vi "Auto_Inspection Station MainS8.vi"(7 "Boolean 2":refnum<vi>, 8 "站別":refnum<vi>, 9 "站別":i32, 10 "ActRef":refnum<vi>, 11 "Station Action.lvclass":refnum<class "Station Action.lvclass">) -> ()   [LabVIEW 2019]
uses:
  Station Class/Station Action.lvclass
  Ctrl/Station Action.ctl
  Ctrl/Auto Inspection Data Name.ctl
  FlowCtrl Class/Ctrl/Auto Inspection_IN Name2.ctl
  FlowCtrl Class/Vision AI/Ctl/S8 Station IO.ctl
  Ctrl/ModbusCmd.ctl
  Function/Main UI/Glb/Main_UI Gb.vi
  LLB/Commonly VI/Main Glb.vi
  Ctrl/Auto Inspection Main UI Ref.ctl
  LLB/Commonly VI.lvlib
  Ctrl/Auto Inspection Station Name2.ctl
panel:
  in  "Boolean":bool
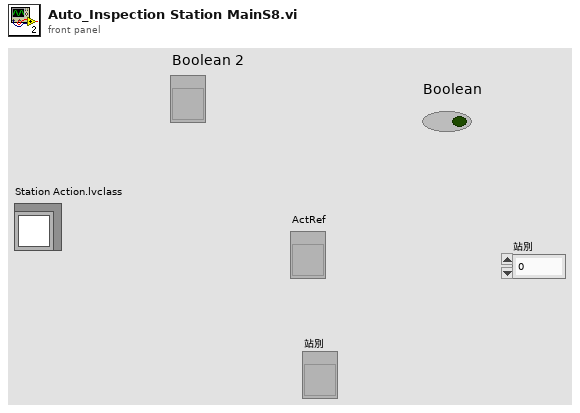
[diagram p1: front panel]
types:
  T1 = typedef "Station Action.ctl" = enum16{"Wait Item In", "Dectect Action", "ImformOut"}
  T2 = cluster{"AutoRunFlg":refnum<vi>, "Action Finish Flg":refnum<vi>, "Remaining Action":refnum<vi>, "Btn_AutoRun":refnum<vi>, "Manual Flg":refnum<vi>, "Sub Process Error":refnum<vi>}
  T3 = typedef "Auto Inspection Data Name.ctl" = enum16{"LocalRun", "ItemSN(TimeCode)", "CurrentAction", "Error", "Data", "OKNG", "電壓值", "電壓值判斷", "電流值", "電流值判斷", "Laser1 Data", "Laser2 Data", "Laser OKNG", "StationNO"}
  T4 = cluster{"starting address":u16, "number of inputs":u16, "Sat Coils":bool[], "Holding Registers":u16[]}
  T5 = typedef "ModbusCmd.ctl" = enum16{"Connect", "Disconnect", "Init", "Fetch Basic Objects", "Fetch Input Refisters", "Fetch Discrete Inputs", "Set Coils", "Set Holding Registers", "Write Single Holding", "Exit"}
  T6 = typedef "Auto Inspection_IN Name2.ctl" = enum16{"S0 Station", "S1 Barcode ", "S2 Tool Format", "S3 Tool Prpgram", "S4 Tool Sacn", "S11 Laser Detect", "S8 Vision AI"}
  T7 = typedef "S8 Station IO.ctl" = enum16{"S8_PC動作中(address 80)", "S8 AI 浪代OK(address 81)", "S8 AI 浪代NG(address 82)", "S8 AI 動作完成"}
  T8 = typedef "Auto Inspection Station Name2.ctl" = enum16{"S1Barcode", "S2Measure", "S3Measure", "S4Measure", "S5Measure", "S11_LaserCheck", "S8_Vision AI"}
  T9 = typedef "Auto Inspection Main UI Ref.ctl" = cluster{"LineScan arrive":refnum<vi>, "LineScanfinish":refnum<vi>, "AI arrive":refnum<vi>, "AI finish":refnum<vi>, "NG Pick arrive":refnum<vi>, "NG Pick finish":refnum<vi>}
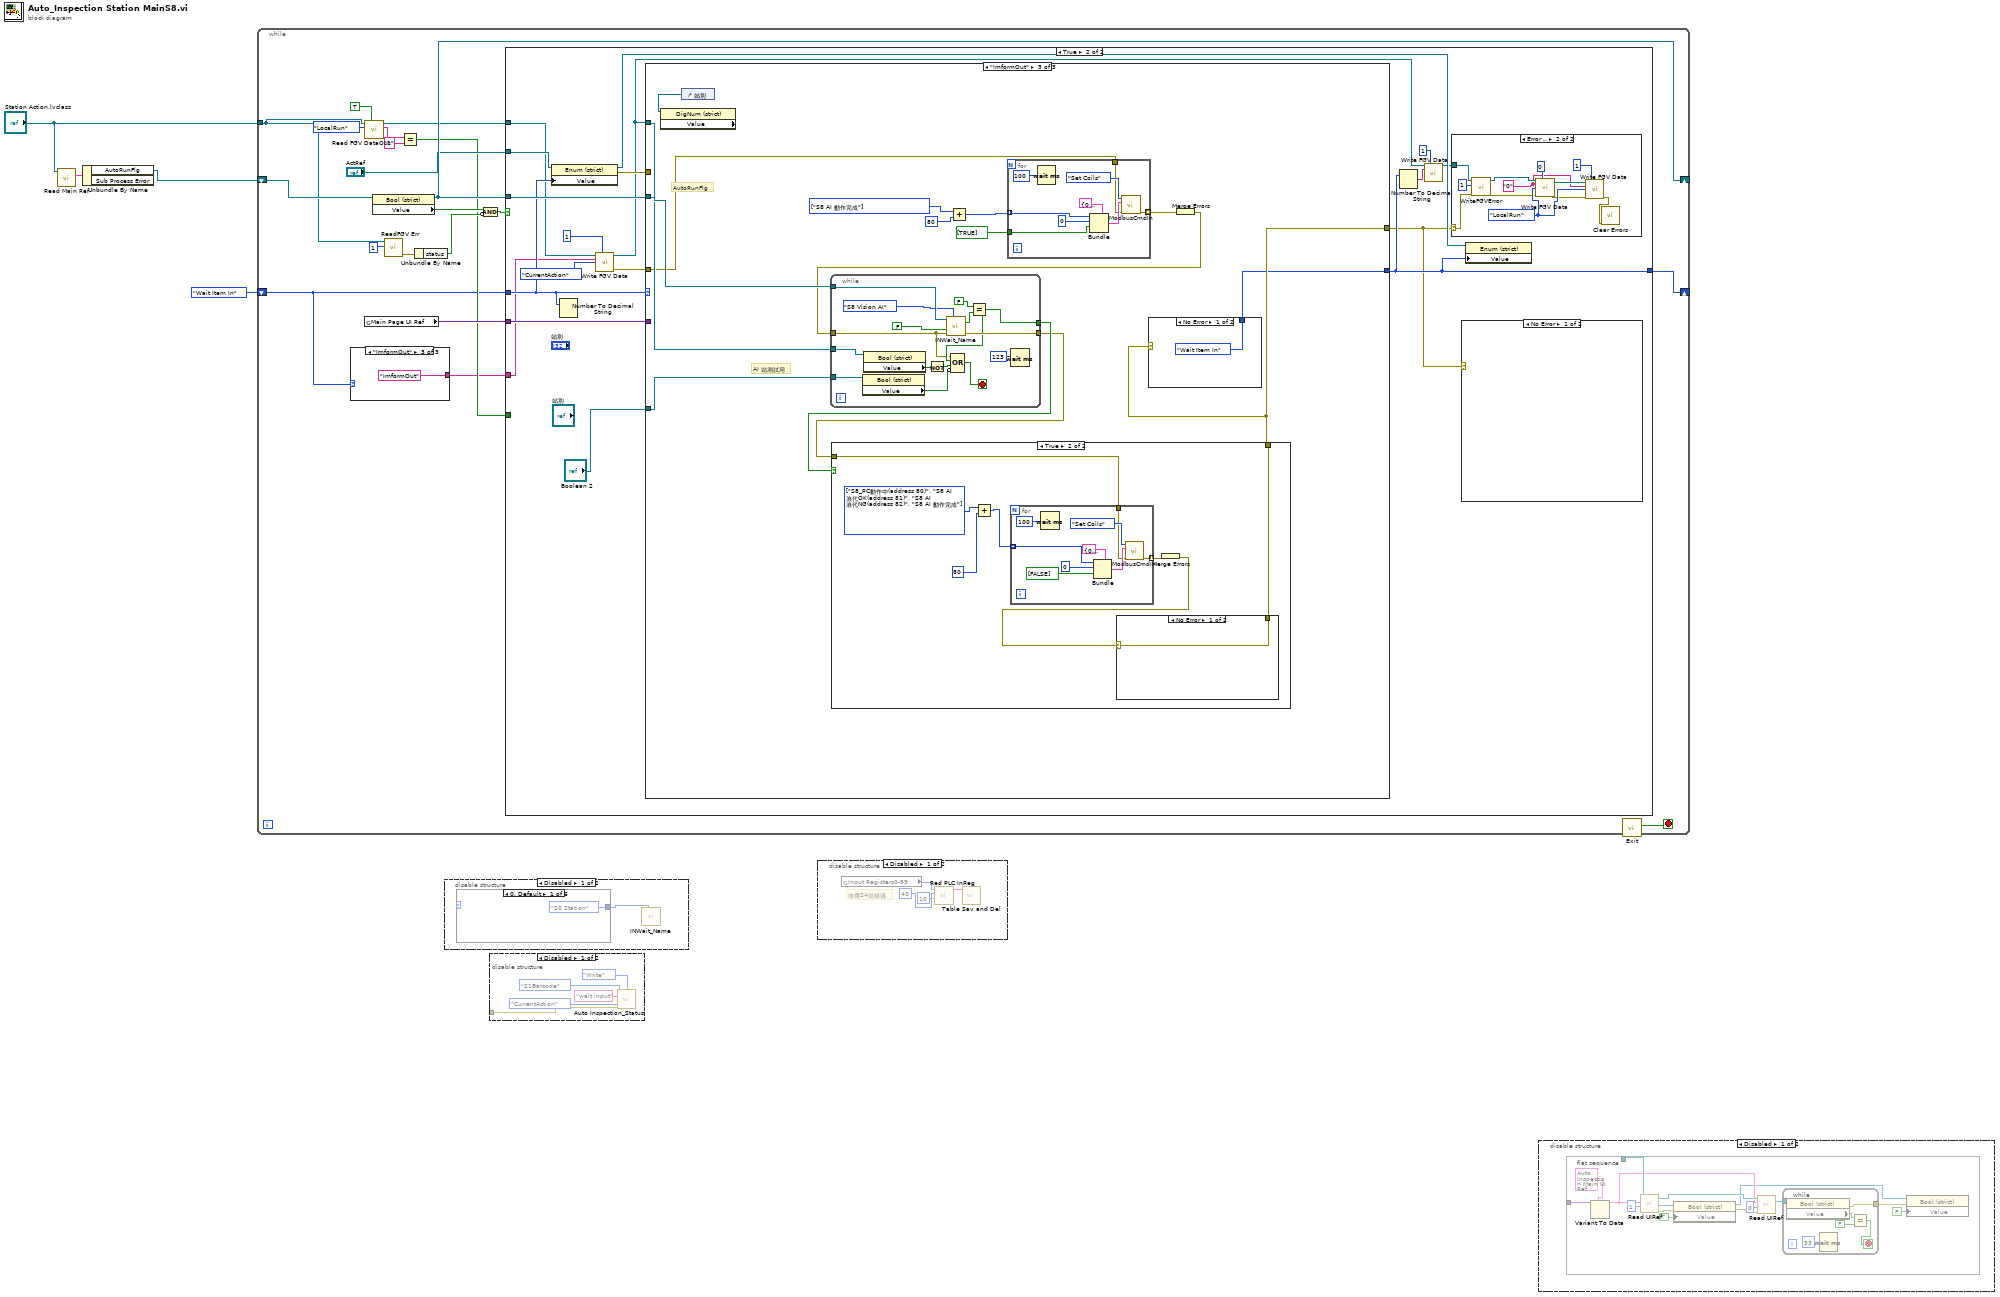
[diagram p0: block diagram]
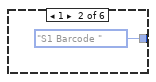
[diagram p3: hidden frame]
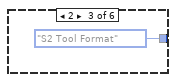
[diagram p4: hidden frame]
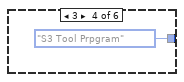
[diagram p5: hidden frame]
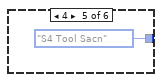
[diagram p6: hidden frame]
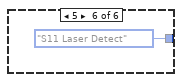
[diagram p7: hidden frame]
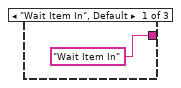
[diagram p11: hidden frame]
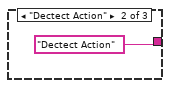
[diagram p12: hidden frame]
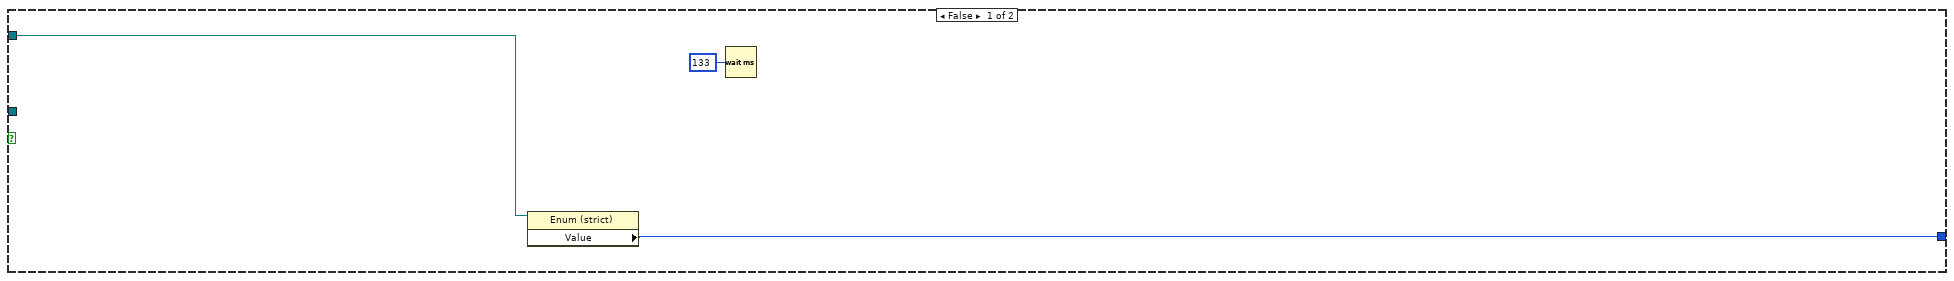
[diagram p13: hidden frame]
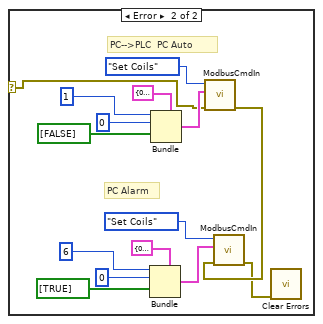
[diagram p14: hidden frame]
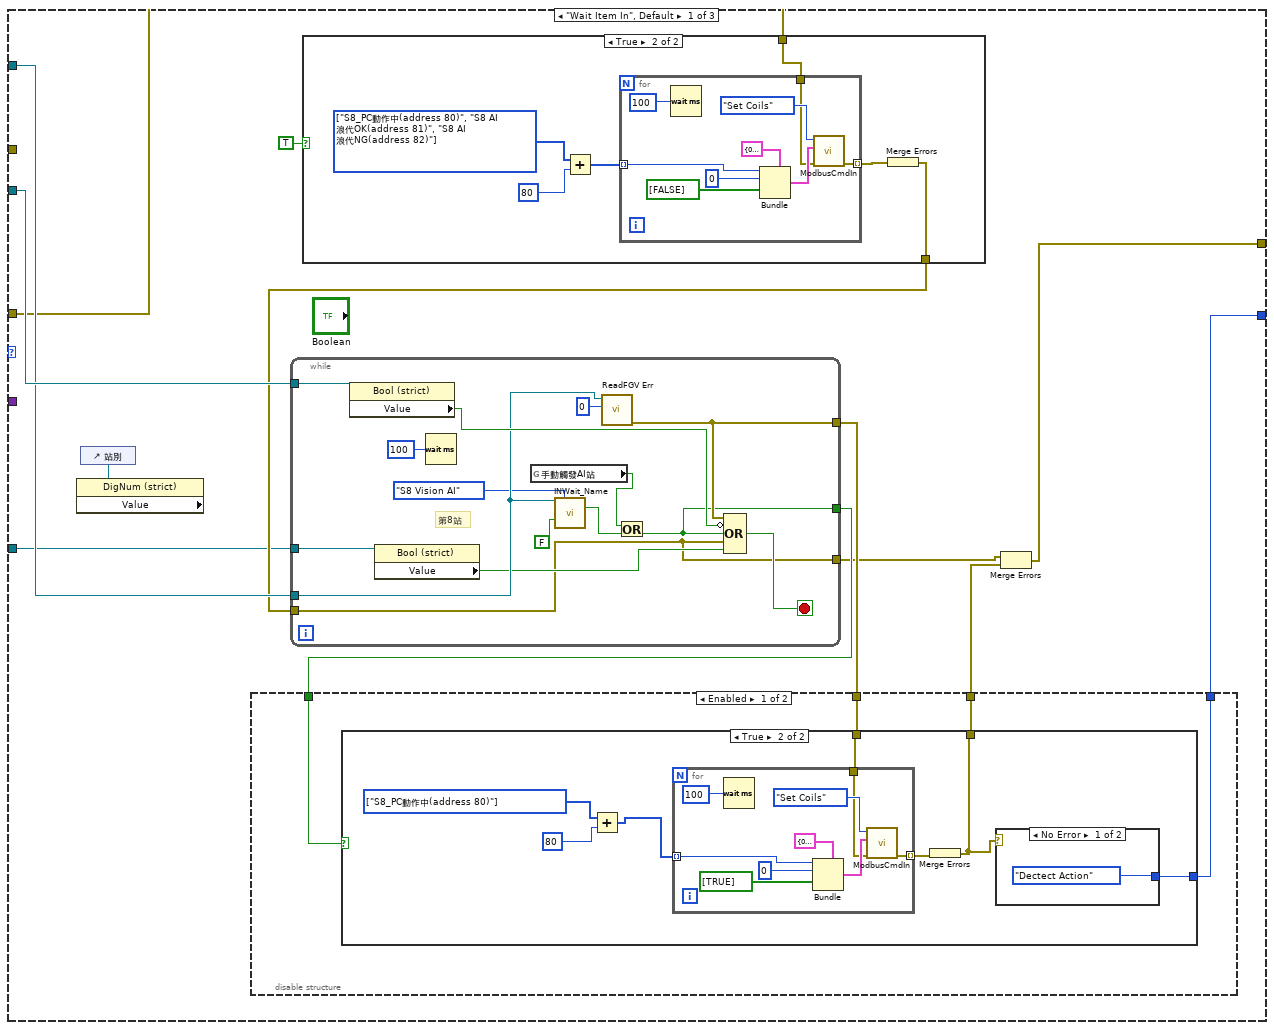
[diagram p16: hidden frame]
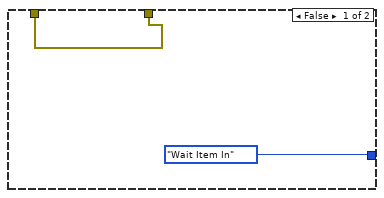
[diagram p17: hidden frame]
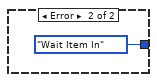
[diagram p18: hidden frame]
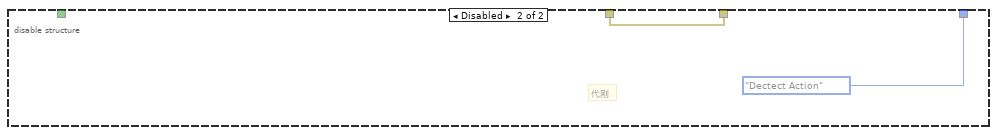
[diagram p19: hidden frame]
diagram:
  n1 = call-dynamic "Read Main Ref.vi"("Main Process Class in"="Station Action.lvclass") -> ("Main Ref"=w3:T2)  [unwired: 8 in, 2 out]
  n2 = Unbundle By Name(w3) -> ("AutoRunFlg"=w1:refnum<vi>)  [unwired: 1 out]
  n3 = while {
    shift-right: [w20] -> _
    shift-left: Station_Action."Wait Item In" -> [w6]
    tunnel: "Station Action.lvclass" -> [w8]
    shift-right: [w18] -> _
    shift-left: w1 -> [w23]
    stop <- w19 stop-if-true
    n4 = case shown="\"ImformOut\"" w6 {
      tunnel: ["Wait Item In" "Dectect Action" "ImformOut"] -> w5
      frame "Wait Item In", Default {
      }
      frame "Dectect Action" {
      }
      frame "ImformOut" {
      }
    }
    n5 = call-dynamic "Read FGV DataOut.vi"("TSt/FConveyor"=TRUE, "Data"=Auto_Inspection_Data_Name."LocalRun", "Station Action in"=w8) -> ("DataOut"=w11:string, "Station Action out"=w14:refnum<class "Station Action.lvclass">)  [unwired: 6 in, 1 out]
    n6 = global read "Main_UI Gb.vi" "Main Page UI Ref"() -> (w21:variant)
    n7 = property class="Bool (strict)"(reference=w23) -> (reference out=w18:refnum<vi>, "Value"=w24:bool)  [unwired: 1 in, 1 out]
    n8 = call-dynamic "ReadFGV Err.vi"("0Cv/1ST"=1, "Station Action in"=w8) -> ("error out"=w16:errorcluster)  [unwired: 8 in, 1 out]
    n9 = Equal?(x=w11, y="1") -> (x = y?=w7:bool)
    n10 = Unbundle By Name(w16) -> ("status"=w15:bool)
    n11 = Compound Arithmetic op=AND(w24, invert w15) -> (w22:bool)
    n12 = case shown="True" w22 {
      tunnel: w18 -> [_ w47]
      tunnel: w6 -> [_ w40]
      tunnel: w21 -> [_ w48]
      tunnel: w14 -> [_ w34]
      tunnel: [w29 w37] -> w20
      tunnel: "ActRef" -> [w30 w46]
      tunnel: w7 -> [_ _]
      tunnel: w5 -> [_ w33]
      frame False {
        n13 = property class="Enum (strict)"(reference=w30) -> ("Value"=w29:T1)  [unwired: 1 in, 2 out]
        n14 = Wait (ms)(milliseconds to wait=u32 133) -> ()  [unwired: 1 out]
      }
      frame True {
        n15 = property class="Enum (strict)"(reference=w46, "Value"=w40) -> (reference out=w45:refnum<vi>, error out=w44:errorcluster)  [unwired: 1 in]
        n16 = Number To Decimal String(number=w40) -> ()  [unwired: 1 in, 1 out]
        n17 = call-dynamic "Write FGV Data.vi"("Station Action in"=w34, "0Cv/1St"=1, "DataIn"=w33, "Data"=Auto_Inspection_Data_Name."CurrentAction") -> ("Station Action out"=w36:refnum<class "Station Action.lvclass">, "error out"=w41:errorcluster)  [unwired: 10 in]
        n18 = case shown="\"ImformOut\"" w40 {
          tunnel: w48 -> [_ _ _]
          tunnel: w36 -> [w87 w148 w165]
          tunnel: w47 -> [w88 _ w164]
          tunnel: [w85 w146 w160] -> w37
          tunnel: w44 -> [_ _ _]
          tunnel: [w77 w147 w161] -> w31
          tunnel: w41 -> [w84 _ w163]
          tunnel: "Boolean 2" -> [w80 _ w151]
          frame "Wait Item In", Default {
            n19 = control-ref of="站別"() -> (w86:refnum<vi>)
            n20 = property class="DigNum (strict)" props=["Value"](reference=w86) -> ()  [unwired: 1 in, 3 out]
            n21 = case shown="True" TRUE {
              tunnel: w84 -> [w115 w121]
              tunnel: [w115 w118] -> w82
              frame False {
                # "代刚"
              }
              frame True {
                w116 = T7[] [enum."S8_PC動作中(address 80)", enum."S8 AI 浪代OK(address 81)", enum."S8 AI 浪代NG(address 82)"] items=["S8_PC動作中(address 80)", "S8 AI 浪代OK(address 81)", "S8 AI 浪代NG(address 82)", "S8 AI 動作完成"]
                n22 = Add(x=w116, y=80) -> (x+y=w120:i32[])
                n23 = for {
                  tunnel: [w124] -> w117 mode=indexing
                  tunnel: w120 -> [w123] mode=indexing
                  tunnel: w121 -> [w122]
                  n24 = Wait (ms)(milliseconds to wait=100) -> ()  [unwired: 1 out]
                  n25 = Bundle(cluster=T4 {"starting address"=0, "number of inputs"=0, "Sat Coils"=[], "Holding Registers"=[]} ("data"), "starting address"=w123, "number of inputs"=u16 0, "Sat Coils"=bool[] [FALSE]) -> (w127:T4)  [unwired: 1 in]
                  n26 = call "ModbusCmdIn.vi"("error in (no error)"=w122, "data"=w127, "Enum"=ModbusCmd."Set Coils") -> ("error out"=w124:errorcluster)  [unwired: 8 in]
                }
                n27 = Merge Errors(w117) -> (w118:errorcluster)
              }
            }
            n28 = while {
              tunnel: [w141] -> w83
              tunnel: w82 -> [w133]
              tunnel: [w132] -> w81
              tunnel: w87 -> [w137]
              tunnel: w88 -> [w138]
              tunnel: w80 -> [w135]
              tunnel: [w133] -> w79
              stop <- w145 stop-if-true
              # "第8站"
              n29 = property class="Bool (strict)"(reference=w138) -> ("Value"=w143:bool)  [unwired: 1 in, 2 out]
              n30 = property class="Bool (strict)"(reference=w135) -> ("Value"=w134:bool)  [unwired: 1 in, 2 out]
              n31 = Wait (ms)(milliseconds to wait=u32 100) -> ()  [unwired: 1 out]
              n32 = global read "Main Glb.vi" "手動觸發AI站"() -> (w131:bool)
              n33 = call "INWait_Name.vi"("FlowCtrl in"=w137, "Input2"=Auto_Inspection_IN_Name2."S8 Vision AI", "Wait?"=FALSE) -> ("StatusOut"=w139:bool)  [unwired: 9 in, 3 out]
              n34 = call-dynamic "ReadFGV Err.vi"("0Cv/1ST"=0, "Station Action in"=w137) -> ("error out"=w141:errorcluster)  [unwired: 8 in, 1 out]
              n35 = Or(x=w131, y=w139) -> (x .or. y?=w132:bool)
              n36 = Compound Arithmetic op=OR(w141, invert w143, w132, w133, w134) -> (w145:bool)
            }
            n37 = disable-structure shown="Enabled" {
              disable-tunnel: [w92 Station_Action."Dectect Action"] -> w85
              disable-tunnel: w83 -> [w91 w114]
              disable-tunnel: w81 -> [w90 _]
              disable-tunnel: [w89 w114] -> w78
              frame Enabled {
                n38 = case shown="True" w90 {
                  tunnel: w91 -> [w93 w98]
                  tunnel: [w93 w97] -> w89
                  tunnel: [Station_Action."Wait Item In" w96] -> w92
                  frame False {
                  }
                  frame True {
                    w95 = T7[] [enum."S8_PC動作中(address 80)"] items=["S8_PC動作中(address 80)", "S8 AI 浪代OK(address 81)", "S8 AI 浪代NG(address 82)", "S8 AI 動作完成"]
                    n39 = Add(x=w95, y=80) -> (x+y=w99:i32[])
                    n40 = for {
                      tunnel: [w106] -> w100 mode=indexing
                      tunnel: w99 -> [w105] mode=indexing
                      tunnel: w98 -> [w104]
                      n41 = Wait (ms)(milliseconds to wait=100) -> ()  [unwired: 1 out]
                      n42 = Bundle(cluster=T4 {"starting address"=0, "number of inputs"=0, "Sat Coils"=[], "Holding Registers"=[]} ("data"), "starting address"=w105, "number of inputs"=u16 0, "Sat Coils"=bool[] [TRUE]) -> (w109:T4)  [unwired: 1 in]
                      n43 = call "ModbusCmdIn.vi"("error in (no error)"=w104, "data"=w109, "Enum"=ModbusCmd."Set Coils") -> ("error out"=w106:errorcluster)  [unwired: 8 in]
                    }
                    n44 = Merge Errors(w100) -> (w97:errorcluster)
                    n45 = case shown="No Error" w97 {
                      tunnel: [Station_Action."Dectect Action" Station_Action."Wait Item In"] -> w96
                      frame No Error {
                      }
                      frame Error {
                      }
                    }
                  }
                }
              }
              frame Disabled {
                # "代刚"
              }
            }
            n46 = Merge Errors(w79, w78) -> (w77:errorcluster)
          }
          frame "Dectect Action" {
            n47 = call-dynamic "Station Detail Main.vi"("Station Action in"=w148) -> ("error out"=w147:errorcluster)  [unwired: 8 in, 2 out]
            n48 = case shown="Error .." w147 {
              tunnel: [Station_Action."ImformOut" ("Station Out") Station_Action."Wait Item In" ("Station Out")] -> w146
              frame No Error {
              }
              frame Error {
              }
            }
          }
          frame "ImformOut" {
            w152 = T7[] [enum."S8 AI 動作完成"] items=["S8_PC動作中(address 80)", "S8 AI 浪代OK(address 81)", "S8 AI 浪代NG(address 82)", "S8 AI 動作完成"]
            # "AI 站測試用"
            # "AutoRunFlg"
            n49 = control-ref of="站別"() -> (w162:refnum<vi>)
            n50 = property class="DigNum (strict)" props=["Value"](reference=w162) -> ()  [unwired: 1 in, 3 out]
            n51 = Add(x=w152, y=80) -> (x+y=w159:i32[])
            n52 = for {
              tunnel: [w171] -> w158 mode=indexing
              tunnel: w163 -> [w170]
              tunnel: w159 -> [w169] mode=indexing
              tunnel: bool[] [TRUE] ("Sat Coils") -> [w168]
              n53 = Wait (ms)(milliseconds to wait=100) -> ()  [unwired: 1 out]
              n54 = Bundle(cluster=T4 {"starting address"=0, "number of inputs"=0, "Sat Coils"=[], "Holding Registers"=[]} ("data"), "starting address"=w169, "number of inputs"=u16 0, "Sat Coils"=w168) -> (w174:T4)  [unwired: 1 in]
              n55 = call "ModbusCmdIn.vi"("error in (no error)"=w170, "data"=w174, "Enum"=ModbusCmd."Set Coils") -> ("error out"=w171:errorcluster)  [unwired: 8 in]
            }
            n56 = Merge Errors(w158) -> (w157:errorcluster)
            n57 = while {
              tunnel: w165 -> [w209]
              tunnel: w164 -> [w208]
              tunnel: [w201] -> w156
              tunnel: [w204] -> w155
              tunnel: w157 -> [w196]
              tunnel: w151 -> [w198]
              stop <- w205 stop-if-true
              n58 = property class="Bool (strict)"(reference=w198) -> ("Value"=w197:bool)  [unwired: 1 in, 2 out]
              n59 = property class="Bool (strict)"(reference=w208) -> ("Value"=w207:bool)  [unwired: 1 in, 2 out]
              n60 = Not(x=w207) -> (.not. x?=w206:bool)
              n61 = call "INWait_Name.vi"("FlowCtrl in"=w209, "Input2"=Auto_Inspection_IN_Name2."S8 Vision AI", "Wait?"=FALSE, "error in (no error)"=w196) -> ("StatusOut"=w203:bool, "error out"=w204:errorcluster)  [unwired: 8 in, 2 out]
              n62 = Equal?(x=FALSE, y=w203) -> (x = y?=w201:bool)
              n63 = Compound Arithmetic op=OR(w196, w201, w206, invert w197) -> (w205:bool)
              n64 = Wait (ms)(milliseconds to wait=123) -> ()  [unwired: 1 out]
            }
            n65 = case shown="True" w156 {
              tunnel: w155 -> [w177 w183]
              tunnel: [w177 w180] -> w161
              frame False {
              }
              frame True {
                w178 = T7[] [enum."S8_PC動作中(address 80)", enum."S8 AI 浪代OK(address 81)", enum."S8 AI 浪代NG(address 82)", enum."S8 AI 動作完成"] items=["S8_PC動作中(address 80)", "S8 AI 浪代OK(address 81)", "S8 AI 浪代NG(address 82)", "S8 AI 動作完成"]
                n66 = Add(x=w178, y=80) -> (x+y=w182:i32[])
                n67 = for {
                  tunnel: w182 -> [w187] mode=indexing
                  tunnel: [w189] -> w184 mode=indexing
                  tunnel: w183 -> [w188]
                  n68 = Wait (ms)(milliseconds to wait=100) -> ()  [unwired: 1 out]
                  n69 = Bundle(cluster=T4 {"starting address"=0, "number of inputs"=0, "Sat Coils"=[], "Holding Registers"=[]} ("data"), "starting address"=w187, "number of inputs"=u16 0, "Sat Coils"=bool[] [FALSE]) -> (w192:T4)  [unwired: 1 in]
                  n70 = call "ModbusCmdIn.vi"("error in (no error)"=w188, "data"=w192, "Enum"=ModbusCmd."Set Coils") -> ("error out"=w189:errorcluster)  [unwired: 8 in]
                }
                n71 = Merge Errors(w184) -> (w181:errorcluster)
                n72 = case shown="No Error" w181 {
                  selector: w181 -> [w185 w186]
                  tunnel: [w185 w186] -> w180
                  frame No Error {
                  }
                  frame Error {
                  }
                }
              }
            }
            n73 = case shown="No Error" w161 {
              tunnel: [Station_Action."Wait Item In" Station_Action."ImformOut"] -> w160
              frame No Error {
              }
              frame Error {
              }
            }
          }
        }
        n74 = Number To Decimal String(number=w37) -> (decimal integer string=w38:string)  [unwired: 1 in]
        n75 = call-dynamic "Write FGV Data.vi"("Station Action in"=w36, "0Cv/1St"=1, "DataIn"=w38) -> ("Station Action out"=w35:refnum<class "Station Action.lvclass">)  [unwired: 11 in, 1 out]
        n76 = case shown="Error .." w31 {
          selector: w31 -> [_ w74]
          tunnel: w35 -> [_ w73]
          frame No Error {
          }
          frame Error {
            w68 = Auto_Inspection_Data_Name."LocalRun" ("Data")
            w65 = "0" ("DataIn")
            n77 = call-dynamic "WriteFGVError.vi"("error in (no error)"=w74, "0Cv/1St"=1, "Station Action in"=w73) -> ("error out"=w66:errorcluster, "Station Action out"=w69:refnum<class "Station Action.lvclass">)  [unwired: 7 in]
            n78 = call-dynamic "Write FGV Data.vi"("Station Action in"=w69, "0Cv/1St"=0, "DataIn"=w65, "Data"=w68, "error in (no error)"=w66) -> ("Station Action out"=w70:refnum<class "Station Action.lvclass">, "error out"=w67:errorcluster)  [unwired: 9 in]
            n79 = call-dynamic "Write FGV Data.vi"("Station Action in"=w70, "0Cv/1St"=1, "DataIn"=w65, "Data"=w68, "error in (no error)"=w67) -> ("error out"=w64:errorcluster)  [unwired: 9 in, 1 out]
            n80 = call <vilib>:"Clear Errors.vi"("error in (no error)"=w64) -> ()  [unwired: 5 in, 2 out]
          }
        }
        n81 = case shown="No Error" w31 {
          selector: w31 -> [_ w50]
          frame No Error {
          }
          frame Error {
            # "PC Alarm"
            # "PC-->PLC  PC Auto"
            n82 = Bundle(cluster=T4 {"starting address"=0, "number of inputs"=0, "Sat Coils"=[], "Holding Registers"=[]} ("data"), "starting address"=6, "number of inputs"=u16 0, "Sat Coils"=bool[] [TRUE]) -> (w57:T4)  [unwired: 1 in]
            n83 = Bundle(cluster=T4 {"starting address"=0, "number of inputs"=0, "Sat Coils"=[], "Holding Registers"=[]} ("data"), "starting address"=1, "number of inputs"=u16 0, "Sat Coils"=bool[] [FALSE]) -> (w58:T4)  [unwired: 1 in]
            n84 = call "ModbusCmdIn.vi"("error in (no error)"=w50, "data"=w58, "Enum"=ModbusCmd."Set Coils") -> ("error out"=w51:errorcluster)  [unwired: 8 in]
            n85 = call "ModbusCmdIn.vi"("error in (no error)"=w51, "data"=w57, "Enum"=ModbusCmd."Set Coils") -> ("error out"=w49:errorcluster)  [unwired: 8 in]
            n86 = call <vilib>:"Clear Errors.vi"("error in (no error)"=w49) -> ()  [unwired: 5 in, 2 out]
          }
        }
        n87 = property class="Enum (strict)"(reference=w45, "Value"=w37) -> ()  [unwired: 1 in, 2 out]
      }
    }
    n88 = call "Exit.vi"() -> ("ExitOut"=w19:bool)  [unwired: 11 in]
  }
  n89 = disable-structure shown="Disabled" {
    frame Disabled {
      n90 = case shown="0, Default" {
        selector: _ -> [_ _ _ _ _ _]
        tunnel: [Auto_Inspection_IN_Name2."S0 Station" Auto_Inspection_IN_Name2."S1 Barcode " Auto_Inspection_IN_Name2."S2 Tool Format" Auto_Inspection_IN_Name2."S3 Tool Prpgram" Auto_Inspection_IN_Name2."S4 Tool Sacn" Auto_Inspection_IN_Name2."S11 Laser Detect"] -> w211
        frame 0, Default {
        }
        frame 1 {
        }
        frame 2 {
        }
        frame 3 {
        }
        frame 4 {
        }
        frame 5 {
        }
      }
      n91 = call "INWait_Name.vi"("Input2"=w211) -> ()  [unwired: 11 in, 4 out]
    }
    frame Enabled {
    }
  }
  n92 = disable-structure shown="Disabled" {
    disable-tunnel: _ -> [w218 _]
    frame Disabled {
      n93 = call "Auto Inspection_Status.vi"("Action"=enum16{"Initial", "Write", "Read"}."Write", "DataIn"="wait input", "Station"=Auto_Inspection_Station_Name2."S1Barcode", "Data"=Auto_Inspection_Data_Name."CurrentAction", "error in"=w218) -> ()  [unwired: 8 in, 3 out]
    }
    frame Enabled {
    }
  }
  n94 = disable-structure shown="Disabled" {
    frame Disabled {
      # "收尋S4站條碼"
      n95 = global read "Main Glb.vi" "Input Registers0-99"() -> (w223:u16[])
      n96 = call "Red PLC InReg.vi"("length"=10, "index"=40, "Input Registers Arr"=w223) -> ("Rad In Reg"=w224:string)  [unwired: 7 in, 1 out]
      n97 = call "Table Sav and Del.vi"("SN"=w224) -> ()  [unwired: 9 in, 2 out]
    }
    frame Enabled {
    }
  }
  n98 = disable-structure shown="Disabled" {
    frame Disabled {
      n99 = flat-sequence {
        tunnel: _ -> [w241]
        tunnel: _ -> [w239]
        frame #0 {
          n100 = Variant To Data(type=T9 {"LineScan arrive"=refnum, "LineScanfinish"=refnum, "AI arrive"=refnum, "AI finish"=refnum, "NG Pick arrive"=refnum, "NG Pick finish"=refnum} ("UI Ref"), Variant=w239) -> (data=w231:T9)  [unwired: 1 in, 1 out]
          n101 = call-dynamic "Read UIRef.vi"("0Arrive/1Finish"=1, "UI Ref"=w231, "Station Action in"=w241) -> ("error out"=w234:errorcluster, "RefOut"=w240:refnum<vi>, "Station Action out"=w235:refnum<class "Station Action.lvclass">)  [unwired: 6 in]
          n102 = property class="Bool (strict)"(reference=w240, error in=w234, "Value"=TRUE) -> (reference out=w228:refnum<vi>, error out=w233:errorcluster)
          n103 = call-dynamic "Read UIRef.vi"("error in (no error)"=w233, "0Arrive/1Finish"=0, "UI Ref"=w231, "Station Action in"=w235) -> ("RefOut"=w230:refnum<vi>)  [unwired: 5 in, 2 out]
          n104 = while {
            tunnel: w230 -> [w247]
            tunnel: [w242] -> w227
            stop <- w246 stop-if-true
            n105 = property on="Property Node" class="Bool (strict)"(reference=w247) -> (error out=w242:errorcluster, "Value"=w245:bool)  [unwired: 1 in, 1 out]
            n106 = Wait (ms)(milliseconds to wait=u32 33) -> ()  [unwired: 1 out]
            n107 = Equal?(x=w245, y=FALSE) -> (x = y?=w246:bool)
          }
          n108 = property class="Bool (strict)"(reference=w228, error in=w227, "Value"=FALSE) -> ()  [unwired: 2 out]
        }
      }
    }
    frame Enabled {
    }
  }
